vi "Solenoid.vi"(8 "Value":T1, 11 "Solenoid":string) -> ()   [LabVIEW 2019]
uses:
  Implementation/Pnuematics Operations.ctl
  Implementation/Pnuematics Setpoints.ctl
  <vilib>/Rock Robotics/WPI/Solenoid/WPI_SolenoidValue.ctl
  <vilib>/Rock Robotics/WPI/Framework/Completion Status.ctl
  <vilib>/Rock Robotics/WPI/Framework/Completion Notifier.ctl
  <vilib>/Rock Robotics/WPI/Framework/Command Status Info.ctl
panel:
  in  "Description":string="Reserve"
  in  "Command Name":string
  out "Command Info":T2
  in  "Command Info 2":T2
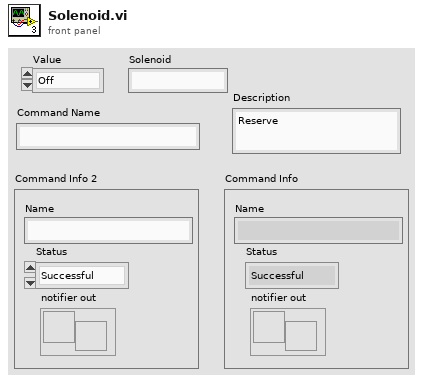
[diagram p1: front panel]
types:
  T1 = typedef "WPI_SolenoidValue.ctl" = enum16{"Off", "On", "Forward", "Reverse"}
  T2 = typedef "Command Status Info.ctl" = cluster{"Name":string, "Status":T3, "notifier out":T4}
  T3 = typedef "Completion Status.ctl" = enum16{"Successful", "Aborted", "Incomplete"}
  T4 = typedef "Completion Notifier.ctl" = refnum<notifier>
  T5 = typedef "Pnuematics Setpoints.ctl" = cluster{"Operation":T6, "Value":T1, "Solenoid":string}
  T6 = typedef "Pnuematics Operations.ctl" = enum16{"Reserve", "CompressorStart", "CompressorStop", "Solenoid", "Read Current", "Immediate"}
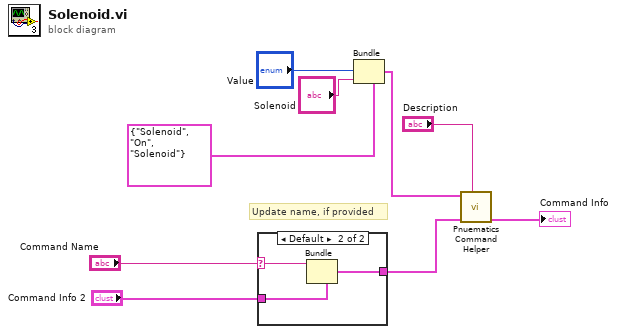
[diagram p0: block diagram]
diagram:
  # "Update name, if provided"
  n1 = case shown="Default" "Command Name" {
    selector: "Command Name" -> [_ w11]
    tunnel: "Command Info 2" -> [w10 w13]
    tunnel: [w10 w12] -> w6
    frame "" {
    }
    frame Default {
      n2 = Bundle(cluster=w13, "Name"=w11) -> (w12:T2)  [unwired: 2 in]
    }
  }
  n3 = Bundle(cluster=T5 {"Operation"=enum."Solenoid", "Value"=enum."On", "Solenoid"="Solenoid"} ("SubSystem Data"), "Value"="Value", "Solenoid"="Solenoid") -> (w3:T5)  [unwired: 1 in]
  n4 = call "Pnuematics Command Helper.vi"("Description"="Description", "Command Info In"=w6, "SubSystem Data"=w3) -> ("Command Info Out"=→"Command Info":T2)  [unwired: 6 in, 2 out]
